vi "TEST - Get Default Data from Variant.vi"(8 "error in (no error)":errorcluster) -> (0 "error out":errorcluster, 2 "Pass":bool)   [LabVIEW 2020, in "test_openg_array.lvlib"]
uses:
  test_openg_array.lvlib
  <userlib>/_OpenG.lib/error/error.llb/openg_error.lvlib
  source/library/openg_variant.lvlib
panel:
  out "Failures":T1(array[cluster])
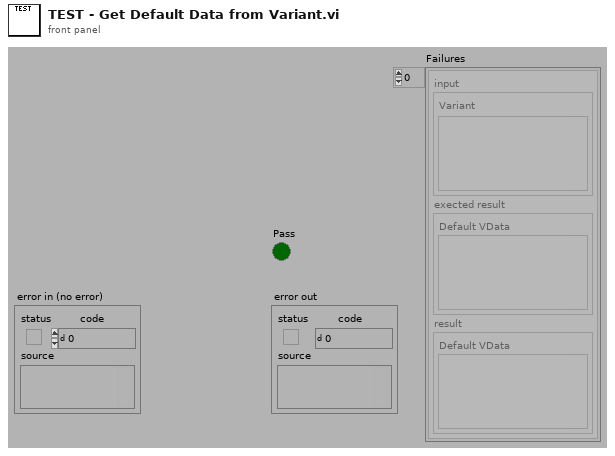
[diagram p1: front panel]
types:
  T1 = cluster{"input":cluster{"Variant":variant}, "exected result":cluster{"Default VData":variant}, "result":cluster{"Default VData":variant}}[]
  T2 = cluster{"input":cluster{"Variant":variant}, "exected result":cluster{"Default VData":variant}, "result":cluster{"Default VData":variant}}
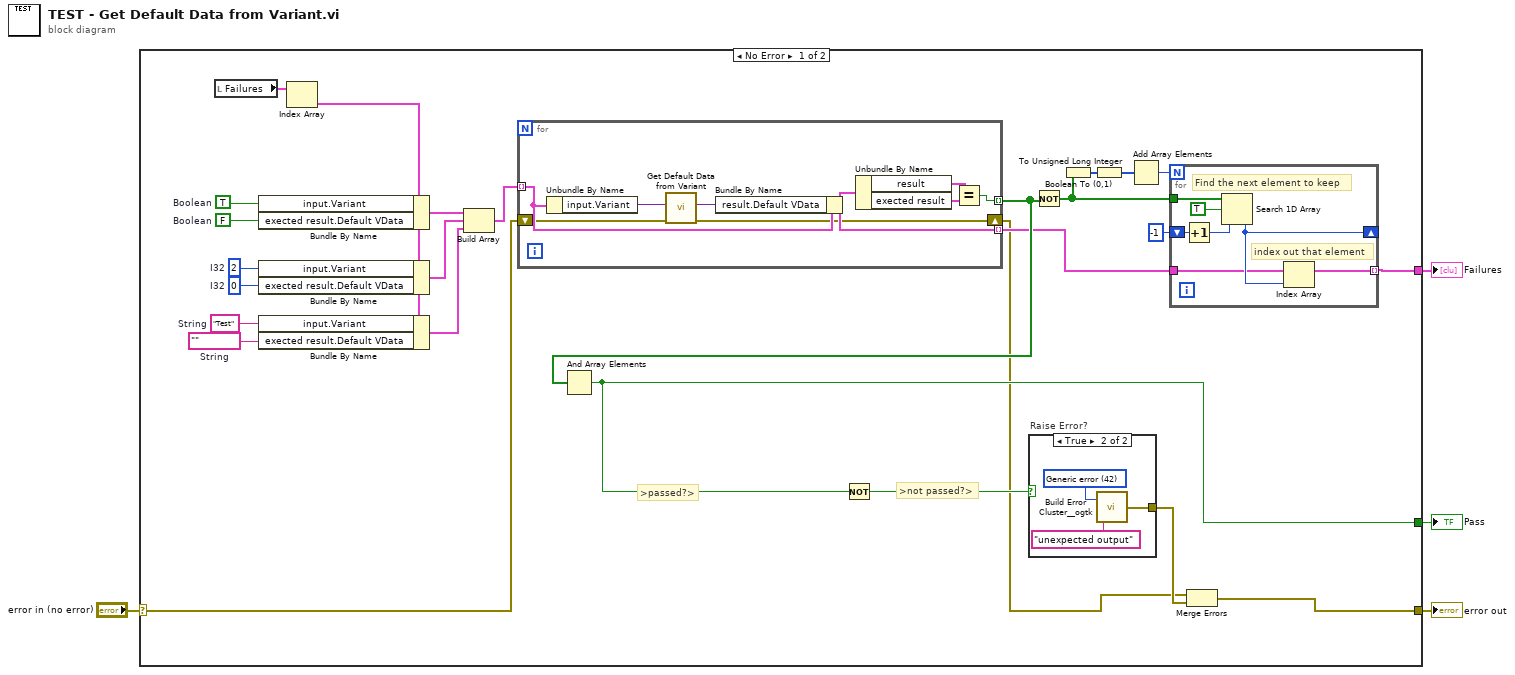
[diagram p0: block diagram]
diagram:
  n1 = case shown="No Error" "error in (no error)" {
    selector: "error in (no error)" -> [w16 w50]
    tunnel: [w27 _] -> w4
    tunnel: [w30 w50] -> w2
    tunnel: [w19 _] -> w1
    frame No Error {
      w5 = ""  # String
      w6 = "Test"  # String
      w9 = 0  # I32
      w10 = 2  # I32
      w13 = FALSE  # Boolean
      w12 = TRUE  # Boolean
      # ">not passed?>"
      # ">passed?>"
      n2 = local read "Failures"() -> (w14:T1)
      n3 = Index Array(array=w14) -> (element=w7:T2)  [unwired: 1 in]
      n4 = Bundle By Name(cluster=w7, "input.Variant"=w12, "exected result.Default VData"=w13) -> (w18:T2)
      n5 = Bundle By Name(cluster=w7, "input.Variant"=w10, "exected result.Default VData"=w9) -> (w11:T2)
      n6 = Bundle By Name(cluster=w7, "input.Variant"=w6, "exected result.Default VData"=w5) -> (w8:T2)
      n7 = Build Array(w18, w11, w8) -> (w17:T1)
      n8 = for {
        tunnel: w17 -> [w45] mode=indexing
        tunnel: [w46] -> w21 mode=indexing
        tunnel: [w44] -> w20 mode=indexing
        shift-right: [w40] -> w15
        shift-left: w16 -> [w39]
        n9 = Unbundle By Name(w45) -> ("input.Variant"=w38:variant)
        n10 = call "Get Default Data from Variant.vi"("error in (no error)"=w39, "Variant"=w38) -> ("error out"=w40:errorcluster, "Default VData"=w41:variant)  [unwired: 8 in]
        n11 = Bundle By Name(cluster=w45, "result.Default VData"=w41) -> (w44:T2)
        n12 = Unbundle By Name(w44) -> ("result"=w43:cluster{"Default VData":variant}, "exected result"=w42:cluster{"Default VData":variant})
        n13 = Equal?(x=w43, y=w42) -> (x = y?=w46:bool)
      }
      n14 = And Array Elements(Boolean array=w21) -> (logical AND=w27:bool)
      n15 = Not(x=w27) -> (.not. x?=w28:bool)
      n16 = case "Raise Error?" shown="True" w28 {
        tunnel: [_ w47] -> w29
        frame False {
        }
        frame True {
          w48 = 42 items=["No error", "Argument error", "Memory is full", "Out of zone", "End of file", "File already open", "Generic file I/O error", "File not found", "File permission error", "Disk is full", "Duplicate path", "Too many files open", "System feature not enabled", "Resource file not found", "Cannot add resource", "Resource not found", "Image not found", "Image memory error", "Pen does not exist", "Config type invalid", "Config token not found", "Config parse error", "Config memory error", "Bad external code format", "Bad external code offset", "External code not present", "Null window", "Destroy window error", "Null menu", "Print aborted", "Bad print record", "Print driver error", "Windows error during printing", "Memory error during printing", "Print dialog error", "Generic print error", "Invalid device refnum", "Device not found", "Device parameter error", "Device unit error", "Cannot open device", "Device call aborted", "Generic error", "Cancelled by user", "Object ID too low", "Object ID too high", "Object not in heap", "Unknown heap", "Unknown object (invalid DefProc)", "Unknown object (DefProc not in table)", "Message out of range", "Invalid (null) method", "Unknown message", "Manager call not supported", "Bad address", "Network operation in progress", "Network operation timed out", "Connection is busy", "Network attribute not supported", "Network error", "Address in use", "System out of memory", "Connection aborted", "Connection refused", "Not connected", "Already connected", "Connection closed", "Initialization error (interapplication manager)", "Bad occurrence", "Wait on unbound occurrence handler", "Occurrence queue overflow", "Datalog type conflict", "Unused", "Unrecognized type (interapplication manager)", "Memory corrupt", "Failed to make temporary DLL", "Old CIN version", "Drag socket not found", "Failed to load drop-object", "Failed to register OLE object", "Failed to release OLE object", "Format specifier type mismatch", "Unknown format specifier", "Too few format specifiers", "Too many format specifiers", "Scan failed", "Newer CIN version", "Error converting to variant", "Runtime menu error", "Password tampered", "Variant attribute not found", "Incompatible variant data type", "Event data is not available", "Event Store is not present", "Occurrence is not found", "Event Queue is not created", "Event info is not available", "Refnum passed is NULL", "Error retrieving Class GUID", "Error retrieving CoClass GUID", "Error retrieving TypeLib GUID.", "Bad built application magic bytes.", "Specific driver is different from the specific driver associated with the Logical Name.", "There is no session opened to the class driver.", "Max Error", "MAX - Error with config objects", "MAX - Error loading configuration", "MAX - Group not supported"]
          n17 = call <userlib>:"Build Error Cluster__ogtk.vi"("String to Prepend to source (\"\")"="unexpected output" ("String to Prepend to source (\"\")"), "code"=w48) -> ("error out"=w47:errorcluster)
        }
      }
      n18 = Not(x=w21) -> (.not. x?=w23:bool[])
      n19 = Boolean To (0,1)(Boolean=w23) -> (0, 1=w24:i16[])
      n20 = To Unsigned Long Integer(number=w24) -> (unsigned 32bit integer=w22:u32[])
      n21 = Add Array Elements(numeric array=w22) -> (sum=w25:u32)
      n22 = for {
        N: w25 -> [_]
        tunnel: w20 -> [w33]
        tunnel: w23 -> [w37]
        shift-right: [w34] -> _
        shift-left: -1 ("start index (0)") -> [w35]
        tunnel: [w32] -> w19 mode=indexing
        # "index out that element"
        # "Find the next element to keep"
        n23 = Increment(x=w35) -> (x+1=w31:i32)
        n24 = Search 1D Array(1D array=w37, element=TRUE, start index (0)=w31) -> (index of element=w34:i32)
        n25 = Index Array(array=w33, index=w34) -> (element=w32:T2)
      }
      n26 = Merge Errors(w15, w29) -> (w30:errorcluster)
    }
    frame Error {
    }
  }
  "Pass" <- w4
  "error out" <- w2
  "Failures" <- w1
